vi "Remove piece.vi"(8 "error in (no error)":errorcluster, 10 "Square":T4={"File"=enum."a", "Rank"=enum."4"}, 11 "Board in":refnum<class "Board.lvclass">) -> (0 "error out":errorcluster, 1 "Removed piece":T1, 3 "Board out":refnum<class "Board.lvclass">)   [LabVIEW 2015, in "Chesslib.lvlib" / "Board.lvclass"]
uses:
  Board.lvclass
  typedef/Square.ctl
  typedef/File.ctl
  typedef/Rank.ctl
  typedef/Piece.ctl
  typedef/Color.ctl
  typedef/Piece type.ctl
  Chesslib.lvlib
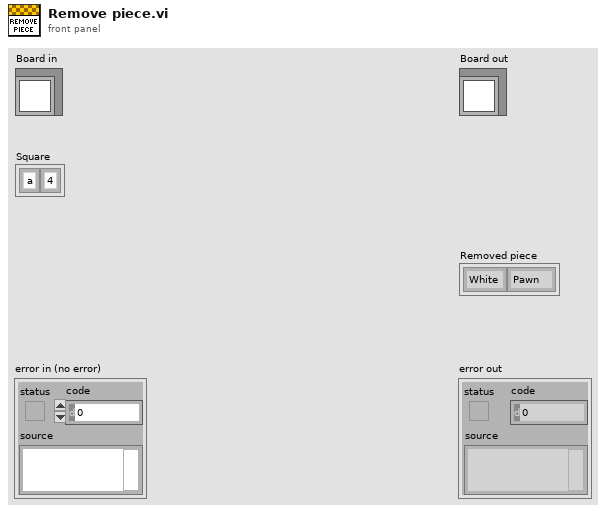
[diagram p1: front panel]
types:
  T1 = typedef "Chesslib.lvlib/Piece.ctl" = cluster{"Color":T2, "Type":T3}
  T2 = typedef "Chesslib.lvlib/Color.ctl" = enum16{"White", "Black"}
  T3 = typedef "Chesslib.lvlib/Piece type.ctl" = enum16{"Pawn", "Bishop", "Knight", "Rook", "Queen", "King"}
  T4 = typedef "Chesslib.lvlib/Square.ctl" = cluster{"File":T5, "Rank":T6}
  T5 = typedef "Chesslib.lvlib/File.ctl" = enum16{"a", "b", "c", "d", "e", "f", "g", "h"}
  T6 = typedef "Chesslib.lvlib/Rank.ctl" = enum16{"1", "2", "3", "4", "5", "6", "7", "8"}
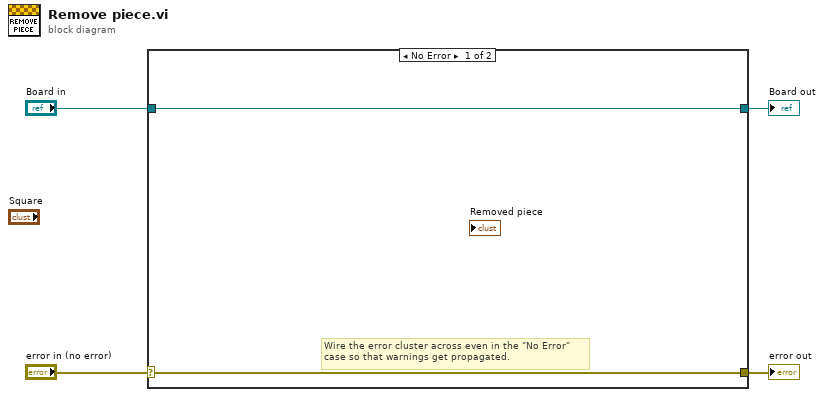
[diagram p0: block diagram]
diagram:
  n1 = case shown="No Error" "error in (no error)" {
    selector: "error in (no error)" -> [w5 w8]
    tunnel: [w5 w8] -> w3
    tunnel: [w6 w7] -> w1
    tunnel: "Board in" -> [w6 w7]
    frame No Error {
      # "Wire the error cluster across even in the \"No Error\"\ncase so that warnings get propagated."
    }
    frame Error {
    }
  }
  "error out" <- w3
  "Board out" <- w1
